vi "Run.vi"(11 "Nav6DevRef":T1) -> ()   [LabVIEW 2014, in "Nav6.lvlib"]
doc: "Reads the data from the Nav6 and makes it availible to the Get VIs.\n\nThe Run VI contains an infinite while loop and should be placed in periodic tasks (similar to the compressor run)."
uses:
  Nav6.lvlib
  Nav6DevRef.ctl
  <vilib>/Rock Robotics/WPI/SerialPort/WPI_SerialPortRef.ctl
  Nav6Mode.ctl
  StopGlobal.vi
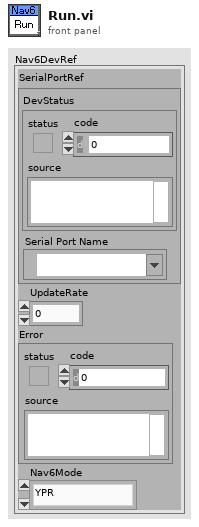
[diagram p1: front panel]
types:
  T1 = typedef "Nav6.lvlib/Nav6DevRef.ctl" = cluster{"SerialPortRef":T2, "UpdateRate":u8, "Error":errorcluster, "Nav6Mode":T3}
  T2 = typedef "WPI_SerialPortRef.ctl" = cluster{"DevStatus":errorcluster, "Serial Port Name":refnum<visa-resource-name>}
  T3 = typedef "Nav6.lvlib/Nav6Mode.ctl" = enum16{"YPR", "Gyro", "Quaternion"}
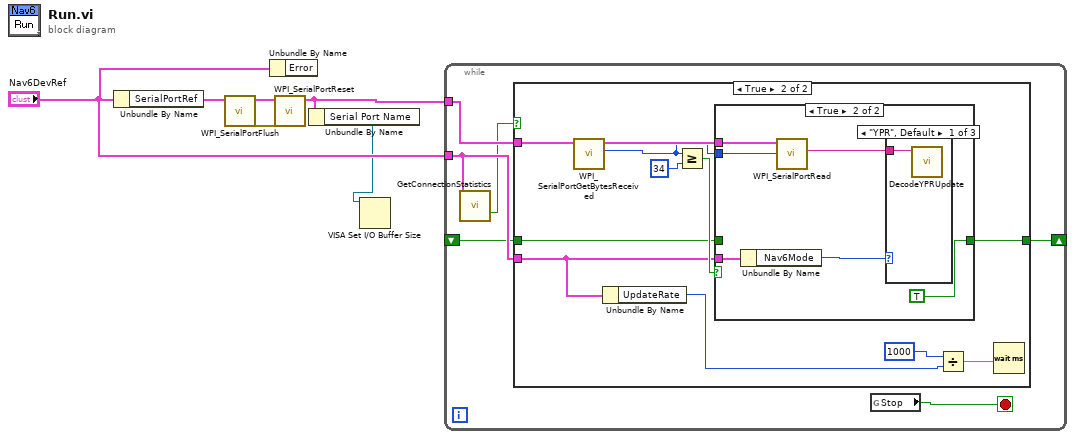
[diagram p0: block diagram]
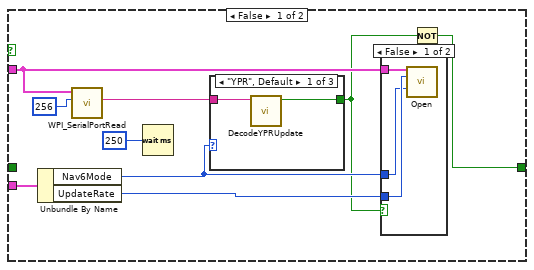
[diagram p2: hidden frame]
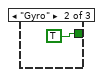
[diagram p4: hidden frame]
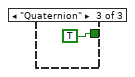
[diagram p5: hidden frame]
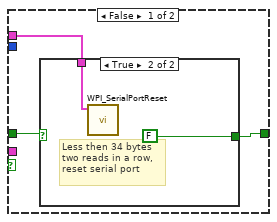
[diagram p6: hidden frame]
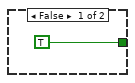
[diagram p7: hidden frame]
diagram:
  n1 = Unbundle By Name("Nav6DevRef") -> ("SerialPortRef"=w4:T2)
  n2 = call <vilib>:"WPI_SerialPortFlush.vi"("SerialPortRef"=w4) -> ("error out"=w6:errorcluster, "SerialPortRef"=w5:T2)  [unwired: 9 in]
  n3 = Unbundle By Name("Nav6DevRef") -> ()  [unwired: 1 out]
  n4 = call <vilib>:"WPI_SerialPortReset.vi"("error in (no error)"=w6, "SerialPortRef"=w5) -> ("SerialPortRef"=w2:T2)  [unwired: 8 in, 1 out]
  n5 = Unbundle By Name(w2) -> ("Serial Port Name"=w1:refnum<visa-resource-name>)
  n6 = VISA Set I/O Buffer Size(VISA resource name=w1) -> ()  [unwired: 3 in, 2 out]
  n7 = while {
    tunnel: w2 -> [w12]
    tunnel: "Nav6DevRef" -> [w10]
    shift-right: [w8] -> _
    shift-left: _ -> [w7]
    stop <- w11 stop-if-true
    n8 = call "GetConnectionStatistics.vi"("Nav6DevRef"=w10) -> ("IsConnected"=w9:bool)  [unwired: 10 in, 4 out]
    n9 = case shown="True" w9 {
      tunnel: w12 -> [w17 w39]
      tunnel: w10 -> [w18 w34]
      tunnel: [w13 w30] -> w8
      tunnel: w7 -> [_ w29]
      frame False {
        n10 = Unbundle By Name(w18) -> ("Nav6Mode"=w15:T3, "UpdateRate"=w16:u8)
        n11 = call <vilib>:"WPI_SerialPortRead.vi"("Num Bytes to Read"=u32 256, "SerialPortRef"=w17) -> ("Buffer"=w20:string)  [unwired: 7 in, 2 out]
        n12 = Wait (ms)(milliseconds to wait=u32 250) -> ()  [unwired: 1 out]
        n13 = case shown="\"YPR\", Default" w15 {
          tunnel: w20 -> [w26 _ _]
          tunnel: [w25 TRUE ("MessageReceived") TRUE ("MessageReceived")] -> w14
          frame "YPR", Default {
            n14 = call "DecodeYPRUpdate.vi"("Buffer"=w26) -> ("MessageReceived"=w25:bool)  [unwired: 10 in]
          }
          frame "Gyro" {
          }
          frame "Quaternion" {
          }
        }
        n15 = case shown="False" w14 {
          tunnel: w17 -> [w24 _]
          tunnel: w16 -> [w23 _]
          tunnel: w15 -> [w22 _]
          frame False {
            n16 = call "Open.vi"("SerialPortRef"=w24, "UpdateRate (100Hz)"=w23, "Nav6Mode (YPR)"=w22) -> ()  [unwired: 6 in, 7 out]
          }
          frame True {
          }
        }
        n17 = Not(x=w14) -> (.not. x?=w13:bool)
      }
      frame True {
        n18 = call <vilib>:"WPI_SerialPortGetBytesReceived.vi"("SerialPortRef"=w39) -> ("Bytes at Port"=w35:u32, "SerialPortRef"=w38:T2)  [unwired: 8 in, 1 out]
        n19 = Unbundle By Name(w34) -> ("UpdateRate"=w32:u8)
        n20 = Greater Or Equal?(x=w35, y=u32 34) -> (x >= y?=w36:bool)
        n21 = case shown="True" w36 {
          tunnel: w34 -> [_ w50]
          tunnel: w38 -> [w41 w48]
          tunnel: w35 -> [_ w47]
          tunnel: [w40 TRUE] -> w30
          tunnel: w29 -> [w42 _]
          frame False {
            n22 = case shown="True" w42 {
              tunnel: w41 -> [_ w45]
              tunnel: [TRUE FALSE] -> w40
              frame False {
              }
              frame True {
                # "Less then 34 bytes \ntwo reads in a row, \nreset serial port"
                n23 = call <vilib>:"WPI_SerialPortReset.vi"("SerialPortRef"=w45) -> ()  [unwired: 9 in, 2 out]
              }
            }
          }
          frame True {
            n24 = Unbundle By Name(w50) -> ("Nav6Mode"=w49:T3)
            n25 = call <vilib>:"WPI_SerialPortRead.vi"("Num Bytes to Read"=w47, "SerialPortRef"=w48) -> ("Buffer"=w51:string)  [unwired: 7 in, 2 out]
            n26 = case shown="\"YPR\", Default" w49 {
              tunnel: w51 -> [w52 _ _]
              frame "YPR", Default {
                n27 = call "DecodeYPRUpdate.vi"("Buffer"=w52) -> ()  [unwired: 10 in, 1 out]
              }
              frame "Gyro" {
              }
              frame "Quaternion" {
              }
            }
          }
        }
        n28 = Divide(x=u32 1000 ("milliseconds to wait"), y=w32) -> (x/y=w31:dbl)
        n29 = Wait (ms)(milliseconds to wait=w31) -> ()  [unwired: 1 out]
      }
    }
    n30 = global read "StopGlobal.vi" "Stop"() -> (w11:bool)
  }
